vi "Rio_Sequence_Selection (DONE).vi"(1 "Sequence Choice":T1) -> (0 "Basic Sequence":T2[](array[typedef]))   [LabVIEW 2017]
uses:
  rio_states.ctl
  radio_buttons_sequence.ctl
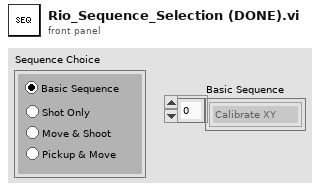
[diagram p1: front panel]
types:
  T1 = typedef "radio_buttons_sequence.ctl" = enum32{"Radio Selection 1", "Radio Selection 2", "Radio Selection 3", "Radio Selection 4"}
  T2 = typedef "rio_states.ctl" = enum16{"Calibrate XY", "Shot Calculation", "Move XY", "Move Theta", "Collect Kicker", "Pickup Kicker", "Retract Kicker", "Hold Kicker", "Kick", "Next Shot", "Stop", "Increment Stage Number", "Increment Coordinate Array", "Wait For Start", "Theta 0", "Reset Encoder"}
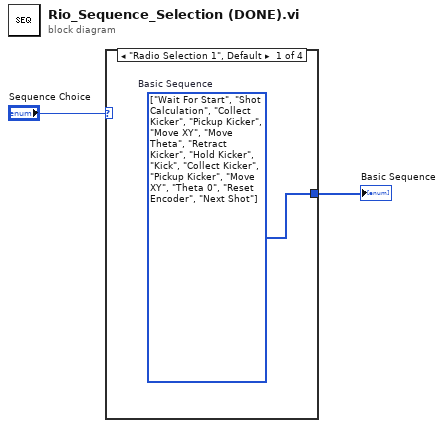
[diagram p0: block diagram]
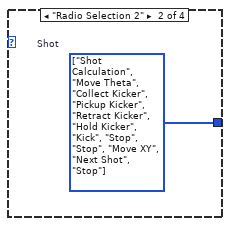
[diagram p2: hidden frame]
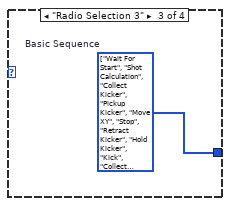
[diagram p3: hidden frame]
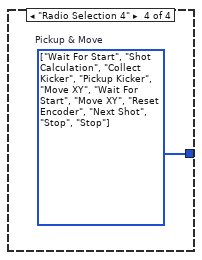
[diagram p4: hidden frame]
diagram:
  n1 = case shown="\"Radio Selection 1\", Default" "Sequence Choice" {
    tunnel: [w3 w4 w5 w6] -> w2
    frame "Radio Selection 1", Default {
      w3 = T2[] [enum."Wait For Start", enum."Shot Calculation", enum."Collect Kicker", enum."Pickup Kicker", enum."Move XY", enum."Move Theta", enum."Retract Kicker", enum."Hold Kicker", enum."Kick", enum."Collect Kicker", enum."Pickup Kicker", enum."Move XY", enum."Theta 0", enum."Reset Encoder", enum."Next Shot"] items=["Calibrate XY", "Shot Calculation", "Move XY", "Move Theta", "Collect Kicker", "Pickup Kicker", "Retract Kicker", "Hold Kicker", "Kick", "Next Shot", "Stop", "Increment Stage Number", "Increment Coordinate Array", "Wait For Start", "Theta 0", "Reset Encoder"]  # Basic Sequence
    }
    frame "Radio Selection 2" {
      w4 = T2[] [enum."Shot Calculation", enum."Move Theta", enum."Collect Kicker", enum."Pickup Kicker", enum."Retract Kicker", enum."Hold Kicker", enum."Kick", enum."Stop", enum."Stop", enum."Move XY", enum."Next Shot", enum."Stop"] items=["Calibrate XY", "Shot Calculation", "Move XY", "Move Theta", "Collect Kicker", "Pickup Kicker", "Retract Kicker", "Hold Kicker", "Kick", "Next Shot", "Stop", "Increment Stage Number", "Increment Coordinate Array", "Wait For Start", "Theta 0", "Reset Encoder"]  # Shot
    }
    frame "Radio Selection 3" {
      w5 = T2[] [enum."Wait For Start", enum."Shot Calculation", enum."Collect Kicker", enum."Pickup Kicker", enum."Move XY", enum."Stop", enum."Retract Kicker", enum."Hold Kicker", enum."Kick", enum."Collect Kicker", enum."Pickup Kicker", enum."Move XY", enum."Theta 0", enum."Next Shot"] items=["Calibrate XY", "Shot Calculation", "Move XY", "Move Theta", "Collect Kicker", "Pickup Kicker", "Retract Kicker", "Hold Kicker", "Kick", "Next Shot", "Stop", "Increment Stage Number", "Increment Coordinate Array", "Wait For Start", "Theta 0", "Reset Encoder"]  # Basic Sequence
    }
    frame "Radio Selection 4" {
      w6 = T2[] [enum."Wait For Start", enum."Shot Calculation", enum."Collect Kicker", enum."Pickup Kicker", enum."Move XY", enum."Wait For Start", enum."Move XY", enum."Reset Encoder", enum."Next Shot", enum."Stop", enum."Stop"] items=["Calibrate XY", "Shot Calculation", "Move XY", "Move Theta", "Collect Kicker", "Pickup Kicker", "Retract Kicker", "Hold Kicker", "Kick", "Next Shot", "Stop", "Increment Stage Number", "Increment Coordinate Array", "Wait For Start", "Theta 0", "Reset Encoder"]  # Pickup & Move
    }
  }
  "Basic Sequence" <- w2
